vi "LTE_DPD_AMPM_EVM_ACP_DL.vi"() -> ()   [LabVIEW 2016]
doc: "This example illustrates how to use the RFmx SpecAn and LTE personalities together with the RFSG drivers to perform AMPM, EVM and ACP measurements with or without digital predistortion (DPD) of the LTE downlink waveform input to the DUT. \n\nDPD is a technique to optimize the operating point of power amplifiers and other non-linear RFIC devices. Power amplifiers are much more efficient if they operate near compression. However, compressing signal amplitudes can significantly deteriorate the amplified signal's quality both, in-band (e.g., EVM increases due to non-linear distortion of the signal's I/Q constellation) and out-of-band (e.g., ACP or SEM test fails due to spectral regrowth). With DPD, the original waveform is first pre-distorted in a way that matches the non-linear effects of the RFIC device before being fed through the device. The resulting output is a much cleaner amplified and/or filtered version of the original waveform. \n\nDifferent DPD models can be used to trade off performance with computational ease, with the Lookup-Table (LUT) model the simplest and the Generalized Memory Polynomial Model (GMP) the most complex. With a LUT, the DPD algorithm achieves gain and phase linearization on average. If you want to correct for memory effects - i.e., an output sample not only depends on the current input but also previous input samples; you will notice that a specific input power value translates into a range of gain and phase values - you would use one of the memory polynomial models. For these models, several parameters such as polynomial order and memory depth are available to fine-tune the model to the DUT behavior."
uses:
  Source/SG/Typedefs/Instrument Configuration.ctl
  <instrlib>/niRFSG/niRFSG.llb/niRFSG Ref Clock Sources.ctl
  Source/Common/Local Oscillator Sharing Mode.ctl
  Source/Common/SA Common Configuration.ctl
  <instrlib>/niRFSG/niRFSG.llb/niRFSG Exported Signal Destinations.ctl
  Source/SA/RFmxLTE/Typedefs/LTE Component Carrier Configuration.ctl
  Source/SA/RFmxLTE/Typedefs/LTE ModAcc Configuration.ctl
  Source/SA/RFmxLTE/Typedefs/LTE ACP Configuration.ctl
  Source/SA/RFmxLTE/Typedefs/LTE ACP Offset Results.ctl
  Source/SA/RFmxLTE/Typedefs/LTE ACP Component Carrier Results.ctl
  Source/SA/RFmxSpecAn/Typedefs/SpecAn AMPM Results.ctl
  Source/SA/RFmxSpecAn/Typedefs/SpecAn AMPM Configuration.ctl
  Source/Common/Waveform.ctl
  Source/Methods/RFmxDPD/Typedefs/Memory Polynomial Configuration.ctl
  Source/Methods/RFmxDPD/Typedefs/Common Configuration.ctl
  Source/SA/RFmxInstr/Typedefs/Instrument Configuration.ctl
  Source/Methods/RFmxDPD/Typedefs/Pre DPD Crest Factor Reduction Configuration.ctl
  Source/Methods/RFmxDPD/Typedefs/Pre DPD Crest Factor Reduction Carrier Channel.ctl
  Source/Methods/RFmxDPD/Typedefs/Apply DPD Crest Factor Reduction Configuration.ctl
  Source/Common/SA Auto Level Configuration.ctl
  <vilib>/RFmx/LTE/mx/RFmxLTE.llb/RFmxLTE ModAcc Fetch EVM per Subcarrier Trace.vi
  <vilib>/RFmx/LTE/mx/RFmxLTE.llb/RFmxLTE ACP Fetch Absolute Powers Trace.vi
  <vilib>/RFmx/LTE/mx/RFmxLTE.llb/RFmxLTE ACP Fetch Relative Powers Trace.vi
  <vilib>/RFmx/LTE/mx/RFmxLTE.llb/RFmxLTE ACP Fetch Spectrum.vi
  <vilib>/RFmx/LTE/mx/RFmxLTE.llb/RFmxLTE ModAcc Fetch PDSCH QPSK Constellation.vi
  <vilib>/RFmx/LTE/mx/RFmxLTE.llb/RFmxLTE ModAcc Fetch PDSCH 64 QAM Constellation.vi
  <vilib>/RFmx/LTE/mx/RFmxLTE.llb/RFmxLTE ModAcc Fetch PDSCH 16 QAM Constellation.vi
  <vilib>/RFmx/LTE/mx/RFmxLTE.llb/RFmxLTE ModAcc Fetch PDSCH 1024 QAM Constellation.vi
  <vilib>/RFmx/LTE/mx/RFmxLTE.llb/RFmxLTE ModAcc Fetch PDSCH 256 QAM Constellation.vi
  <vilib>/RFmx/SpecAn/mx/RFmxSpecAn.llb/RFmxSpecAn AMPM Fetch AM to PM Trace.vi
  <vilib>/RFmx/SpecAn/mx/RFmxSpecAn.llb/RFmxSpecAn AMPM Fetch AM to AM Trace.vi
  Source/SG/SG.lvlib
  Source/SA/RFmxLTE/RFmxLTE.lvlib
  Source/SA/RFmxSpecAn/RFmxSpecAn.lvlib
  Source/Methods/RFmxDPD/RFmxDPD.lvlib
  Source/SA/RFmxInstr/RFmxInstr.lvlib
  Source/Common/Common.lvlib
panel:
  in  "Error Tab Control":enum32{"Page 1", "Page 2"}(tab)
  out "error out":errorcluster
  in  "Display Tab Control":T1(tab)
  out "AM to PM Plot":T2(graph)
  out "AM to AM Plot":T3(graph)
  out "AMPM Measurement Results":T4 {"AM to PM Residual (deg)" format="%.2f"; "AM to AM Residual (dB)" format="%.2f"; "Mean RMS EVM (%)" format="%.2f"; "1 dB Compression Point (dBm)" format="%.2f"; "Mean Linear Gain (dB)" format="%.2f"}
  out "PDSCH QPSK Constellation Trace":cluster{"DMRS  Constellation":csg[]}[](graph)
  out "PDSCH 64 QAM Constellation Trace":cluster{"DMRS  Constellation":csg[]}[](graph)
  out "PDSCH 16 QAM Constellation Trace":cluster{"DMRS  Constellation":csg[]}[](graph)
  out "PDSCH 256 QAM Constellation Trace":cluster{"DMRS  Constellation":csg[]}[](graph)
  out "PDSCH 1024 QAM Constellation Trace":cluster{"DMRS  Constellation":csg[]}[](graph)
  out "EVM Per Subcarrier Trace":cluster{"x0":dbl, "dx":dbl, "y":sgl[]}(graph)
  out "ModAcc Results":T5
  out "ACP Results":T8
  out "Spectrum":cluster{"x0":dbl, "dx":dbl, "y":sgl[]}[](graph)
  out "Reference Waveform":cluster{"t0":dbl, "dt":dbl, "y":sgl[]}(graph)
  in  "Measurement Settings Tab Control":T9(tab)
  in  "RFmx SpecAn AMPM Configuration":T10={"Measurement Interval (s)"=0.0001, "DUT Average Input Power (dBm)"=-20.0, "Signal Type"=0, "Averaging Enabled"=0, "Averaging Count"=10, "Reference Waveform"={"Name"="Wfm", "Data"=refnum, "Signal Bandwidth (Hz)"=0.0, "PAPR (dB)"=0.0, "Burst Length (s)"=0.0, "Sample Rate"=0.0, "Burst Start Locations"=[], "Burst Stop Locations"=[], "Idle Duration Present?"=FALSE, "Runtime Scaling"=0.0, "Script"=""}} {"Reference Waveform"."Runtime Scaling" format="%#_6p"; "Reference Waveform"."Sample Rate" format="%#_6p"; "Reference Waveform"."Burst Length (s)" format="%#_6p"; "Reference Waveform"."PAPR (dB)" format="%.2f"; "Reference Waveform"."Signal Bandwidth (Hz)" format="%#_6p"; "Averaging Enabled" items=["False", "True"]; "Signal Type" items=["Modulated", "Tones"]; "DUT Average Input Power (dBm)" format="%.2f"; "Measurement Interval (s)" format="%.2p"}
  in  "Enable DPD":bool=TRUE
  in  "Common DPD Configuration":T12={"Measurement Interval (s)"=0.0001, "Signal Type"=0, "DUT Average Input Power (dBm)"=-15.0, "Synchronization Method"=1} {"Synchronization Method" items=["Direct"=1, "Alias Protected"=2]; "DUT Average Input Power (dBm)" format="%.2f"; "Signal Type" items=["Modulated", "Tones"]; "Measurement Interval (s)" format="%#.2p"}
  in  "Memory Polynomial Configuration":T13={"Correction Type"=0, "Number of Iterations"=1, " Order"=3, " Depth"=2, "Lead Order"=2, "Lag Order"=2, "Lead Memory Depth"=2, "Lag Memory Depth"=2, "Maximum Lead"=2, "Maximum Lag"=2} {"Number of Iterations" min=1; "Correction Type" items=["Magnitude and Phase", "Magnitude Only", "Phase Only"]}
  in  "Pre DPD Crest Factor Reduction":T14={"Enabled"=0, "Method"=0, "Max Iterations"=10, "Target PAPR (dB)"=8.0, "Shaping Factor"=5.0, "Shaping Threshold (dB)"=-5.0, "Window Type"=7, "Window Length"=10, "Filter Enabled"=0, "Carrier Channels"=[{"Offset (Hz)"=0.0, "Bandwidth (Hz)"=20000000.0}]} {"Carrier Channels"."Bandwidth (Hz)" format="%.2p"; "Carrier Channels"."Offset (Hz)" format="%.2p"; "Filter Enabled" items=["False", "True"]; "Window Type" items=["Flat Top"=1, "Hanning"=2, "Hamming"=3, "Gaussian"=4, "Blackman"=5, "Blackman-Harris"=6, "Kaiser-Bessel"=7]; "Method" items=["Clipping", "Peak Windowing", "Sigmoid"]; "Enabled" items=["False", "True"]}
  in  "Apply DPD Crest Factor Reduction":T16={"Enabled"=0, "Method"=0, "Max Iterations"=10, "Target PAPR Type"=0, "Target PAPR (dB)"=8.0, "Window Type"=7, "Window Length"=10, "Shaping Factor"=5.0, "Shaping Threshold (dB)"=-5.0} {"Target PAPR Type" items=["Input PAPR", "Custom"]; "Window Type" items=["Flat Top"=1, "Hanning"=2, "Hamming"=3, "Gaussian"=4, "Blackman"=5, "Blackman-Harris"=6, "Kaiser-Bessel"=7]; "Method" items=["Clipping", "Peak Windowing", "Sigmoid"]; "Enabled" items=["False", "True"]}
  in  "ModAcc Configuration":T17={"Synchronization Mode"=0, "Measurement Offset"=0, "Measurement Length"=1, "EVM Unit"=0, "Averaging Enabled"=0, "Averaging Count"=10} {"Averaging Enabled" items=["False", "True"]; "EVM Unit" items=["Percentage", "dB"]; "Synchronization Mode" items=["Frame", "Slot", "Marker"]}
  in  "ACP Configuration":T18={"Number of GSM Offsets"=0, "Number of UTRA Offsets"=2, "Number of EUTRA Offsets"=1, "Sweep Time Auto"=1, "Sweep Time Interval (s)"=0.001, "Averaging Enabled"=0, "Averaging Count"=10, "Averaging Type"=0, "RBW Auto"=1, "RBW (Hz)"=30000.0, "RBW Filter Type"=0} {"RBW Filter Type" items=["FFT Based", "Gaussian", "Flat"]; "RBW Auto" items=["False", "True"]; "Averaging Type" items=["RMS", "Log", "Scalar", "Max", "Min"]; "Averaging Enabled" items=["False", "True"]; "Sweep Time Auto" items=["False", "True"]}
  in  "Center Frequency (Hz)":dbl=1950000000.0 format="%.6p"
  in  "Resource Control":enum32{"RFSG", "RFSA", "LTE Signal"}(tab)
  in  "RFSG Resource Name":refnum<k15>="5840"
  in  "Reference Waveform File Path":path=path "C:/Users/Public/Documents/National Instruments/RFIC Test Software/Waveforms/LTE_FDD_DL_1x20MHz_TM11_OS4.tdms"
  in  "SG Configuration":T19={"SelectedPorts"="", "Reference Clock Source"="PXI_CLK", "Carrier Frequency (Hz)"=1000000000.0, "DUT Average Input Power (dBm)"=-10.0, "External Attenuation (dB)"=0.0, "LO Sharing Mode"=enum."Automatic"}
  in  "Marker Event Output Terminal":T22="PXI_Trig0"
  in  "RFSA Resource Name":refnum<k15>="5840"
  in  "Common Configuration":T23={"Center Frequency (Hz)"=1000000000.0, "Reference Level (dBm)"=0.0, "External Attenuation (dB)"=0.0, "Trigger Enabled"=TRUE, "Digital Trigger Source"="PXI_Trig0", "Trigger Delay (s)"=0.0, "Selected Ports"=""} {"Trigger Delay (s)" format="%.2p"; "External Attenuation (dB)" format="%.2f"; "Reference Level (dBm)" format="%.2f"; "Center Frequency (Hz)" format="%.6p"}
  in  "Instrument Configuration":T24={"LO Sharing Mode"=enum."Automatic", "Frequency Reference Source"="PXI_Clk"}
  in  "Auto Level Configuration":T25={"Enabled"=TRUE, "Measurement Interval (s)"=0.01} {"Measurement Interval (s)" min=1e-06 max=100.0 format="%.2p"}
  in  "Signal Configuration":T27={"Link Direction"=0, "Duplex Scheme"=0, "Uplink Downlink Config"=0, "Band"=1, "PUSCH Auto Resource Block Detection Enabled"=1, "Auto DMRS Detection Enabled"=0, "Downlink Auto Cell ID Detection Enabled"=1, "Component Carrier Configurations"=[{"Bandwidth (Hz)"=20000000.0, "Cell ID"=0, "PUSCH Modulation Type"=0, "PUSCH Resource Block Offset"=0, "PUSCH Number of Resource Blocks"=-1, "Downlink Test Model"=0}]} {"Downlink Auto Cell ID Detection Enabled" items=["False", "True"]; "Link Direction" items=["Downlink", "Uplink"]; "Auto DMRS Detection Enabled" items=["False", "True"]; "PUSCH Auto Resource Block Detection Enabled" items=["False", "True"]; "Component Carrier Configurations"."Downlink Test Model" items=["TM1.1", "TM1.2", "TM2", "TM 2a", "TM 3.1", "TM 3.2", "TM 3.3", "TM 3.1a"]; "Component Carrier Configurations"."PUSCH Modulation Type" items=["QPSK", "16 QAM", "64 QAM", "256 QAM", "1024 QAM"]; "Component Carrier Configurations"."Bandwidth (Hz)" items=["200.0 k"=200000.0, "1.4 M"=1400000.0, "3.0 M"=3000000.0, "5.0 M"=5000000.0, "10.0 M"=10000000.0, "15.0 M"=15000000.0, "20.0 M"=20000000.0]; "Uplink Downlink Config" items=["0", "1", "2", "3", "4", "5", "6"]; "Duplex Scheme" items=["FDD", "TDD", "LAA"]}
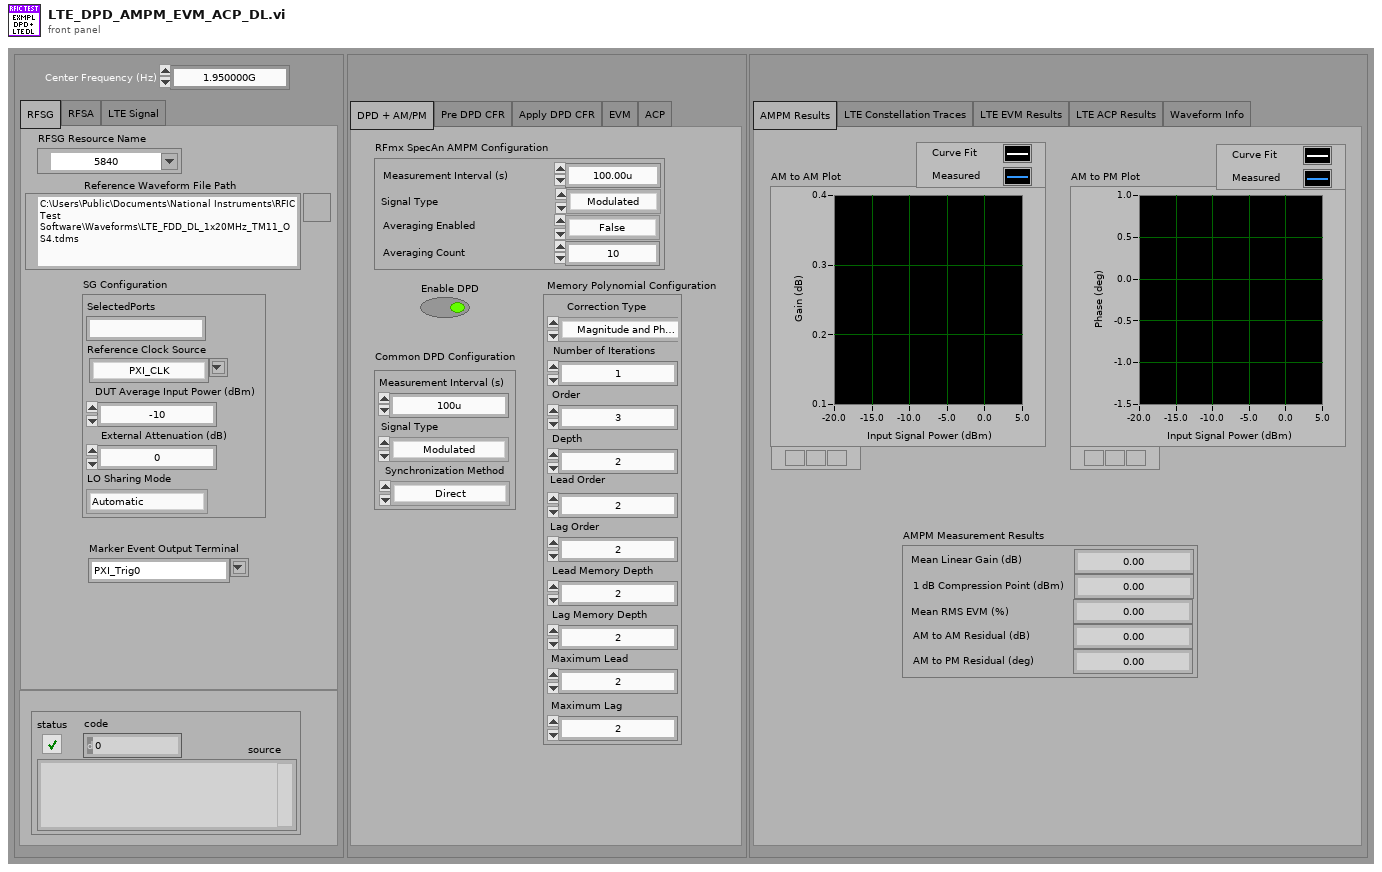
[diagram p1: front panel]
types:
  T1 = enum32{"AMPM Results", "LTE Constellation Traces", "LTE EVM Results", "LTE ACP Results", "Waveform Info"}
  T2 = cluster{"Input Powers (dBm)":sgl[], "Curve Fit AM to PM (dB)":sgl[]}[]
  T3 = cluster{"Input Powers (dBm)":sgl[], "Curve Fit AM to AM (dB)":sgl[]}[]
  T4 = typedef "RFmxSpecAn.lvlib/SpecAn AMPM Results.ctl" = cluster{"Mean Linear Gain (dB)":dbl, "1 dB Compression Point (dBm)":dbl, "Mean RMS EVM (%)":dbl, "AM to AM Residual (dB)":dbl, "AM to PM Residual (deg)":dbl}
  T5 = cluster{"Component Carrier Results":cluster{"Peak Composite EVM Subcarrier Index":i32, "Peak Composite EVM Symbol Index":i32, "Mean RMS Composite EVM":dbl, "Max Peak Composite EVM":dbl, "Mean Frequency Error (Hz)":dbl, "Peak Composite EVM Slot Index":i32}[]}
  T6 = typedef "RFmxLTE.lvlib/LTE ACP Offset Results.ctl" = cluster{"Lower Absolute Power (dBm)":dbl, "Upper Absolute Power (dBm)":dbl, "Lower Relative Power (dB)":dbl, "Upper Relative Power (dB)":dbl, "Frequency (Hz)":dbl, "Integration Bandwidth (Hz)":dbl}
  T7 = typedef "RFmxLTE.lvlib/LTE ACP Component Carrier Results.ctl" = cluster{"Absolute Power (dBm)":dbl, "Relative Power (dB)":dbl}
  T8 = cluster{"Offset Results":T6[], "Component Carrier Results":T7[]}
  T9 = enum32{"DPD + AM/PM", "Pre DPD CFR", "Apply DPD CFR", "EVM", "ACP"}
  T10 = typedef "RFmxSpecAn.lvlib/SpecAn AMPM Configuration.ctl" = cluster{"Measurement Interval (s)":dbl, "DUT Average Input Power (dBm)":dbl, "Signal Type":i32, "Averaging Enabled":i32, "Averaging Count":i32, "Reference Waveform":T11}
  T11 = typedef "Common.lvlib/Waveform.ctl" = cluster{"Name":string, "Data":refnum<data-value>, "Signal Bandwidth (Hz)":dbl, "PAPR (dB)":dbl, "Burst Length (s)":dbl, "Sample Rate":dbl, "Burst Start Locations":i32[], "Burst Stop Locations":i32[], "Idle Duration Present?":bool, "Runtime Scaling":dbl, "Script":string}
  T12 = typedef "RFmxDPD.lvlib/Common Configuration.ctl" = cluster{"Measurement Interval (s)":dbl, "Signal Type":i32, "DUT Average Input Power (dBm)":dbl, "Synchronization Method":i32}
  T13 = typedef "RFmxDPD.lvlib/Memory Polynomial Configuration.ctl" = cluster{"Correction Type":i32, "Number of Iterations":i32, " Order":i32, " Depth":i32, "Lead Order":i32, "Lag Order":i32, "Lead Memory Depth":i32, "Lag Memory Depth":i32, "Maximum Lead":i32, "Maximum Lag":i32}
  T14 = typedef "RFmxDPD.lvlib/Pre DPD Crest Factor Reduction Configuration.ctl" = cluster{"Enabled":i32, "Method":i32, "Max Iterations":i32, "Target PAPR (dB)":dbl, "Shaping Factor":dbl, "Shaping Threshold (dB)":dbl, "Window Type":i32, "Window Length":i32, "Filter Enabled":i32, "Carrier Channels":T15[]}
  T15 = typedef "RFmxDPD.lvlib/Pre DPD Crest Factor Reduction Carrier Channel.ctl" = cluster{"Offset (Hz)":dbl, "Bandwidth (Hz)":dbl}
  T16 = typedef "RFmxDPD.lvlib/Apply DPD Crest Factor Reduction Configuration.ctl" = cluster{"Enabled":i32, "Method":i32, "Max Iterations":i32, "Target PAPR Type":i32, "Target PAPR (dB)":dbl, "Window Type":i32, "Window Length":i32, "Shaping Factor":dbl, "Shaping Threshold (dB)":dbl}
  T17 = typedef "RFmxLTE.lvlib/LTE ModAcc Configuration.ctl" = cluster{"Synchronization Mode":i32, "Measurement Offset":i32, "Measurement Length":i32, "EVM Unit":i32, "Averaging Enabled":i32, "Averaging Count":i32}
  T18 = typedef "RFmxLTE.lvlib/LTE ACP Configuration.ctl" = cluster{"Number of GSM Offsets":i32, "Number of UTRA Offsets":i32, "Number of EUTRA Offsets":i32, "Sweep Time Auto":i32, "Sweep Time Interval (s)":dbl, "Averaging Enabled":i32, "Averaging Count":i32, "Averaging Type":i32, "RBW Auto":i32, "RBW (Hz)":dbl, "RBW Filter Type":i32}
  T19 = typedef "SG.lvlib/Instrument Configuration.ctl" = cluster{"SelectedPorts":string, "Reference Clock Source":T20, "Carrier Frequency (Hz)":dbl, "DUT Average Input Power (dBm)":dbl, "External Attenuation (dB)":dbl, "LO Sharing Mode":T21}
  T20 = typedef "niRFSG Ref Clock Sources.ctl" = string
  T21 = typedef "Common.lvlib/Local Oscillator Sharing Mode.ctl" = enum16{"Automatic", "None"}
  T22 = typedef "niRFSG Exported Signal Destinations.ctl" = string
  T23 = typedef "Common.lvlib/SA Common Configuration.ctl" = cluster{"Center Frequency (Hz)":dbl, "Reference Level (dBm)":dbl, "External Attenuation (dB)":dbl, "Trigger Enabled":bool, "Digital Trigger Source":string, "Trigger Delay (s)":dbl, "Selected Ports":string}
  T24 = typedef "RFmxInstr.lvlib/Instrument Configuration.ctl" = cluster{"LO Sharing Mode":T21, "Frequency Reference Source":string}
  T25 = typedef "Common.lvlib/SA Auto Level Configuration.ctl" = cluster{"Enabled":bool, "Measurement Interval (s)":dbl}
  T26 = typedef "RFmxLTE.lvlib/LTE Component Carrier Configuration.ctl" = cluster{"Bandwidth (Hz)":dbl, "Cell ID":i32, "PUSCH Modulation Type":i32, "PUSCH Resource Block Offset":i32, "PUSCH Number of Resource Blocks":i32, "Downlink Test Model":i32}
  T27 = cluster{"Link Direction":i32, "Duplex Scheme":i32, "Uplink Downlink Config":i32, "Band":i32, "PUSCH Auto Resource Block Detection Enabled":i32, "Auto DMRS Detection Enabled":i32, "Downlink Auto Cell ID Detection Enabled":i32, "Component Carrier Configurations":T26[]}
  T28 = enum16{"ACP", "CHP", "ModAcc", "OBW", "SEM", "PVT", "SlotPhase", "SlotPower"}[]
  T29 = enum16{"ACP", "CCDF", "CHP", "FCnt", "Harmonics", "OBW", "SEM", "Spectrum", "Spur", "TXP", "AMPM", "DPD", "IQ", "IM", "NF", "PhaseNoise", "PAVT"}[]
  T30 = cluster{"Reference Powers (dBm)":sgl[], "Curve Fit AM to AM (dB)":sgl[]}
  T31 = cluster{"Reference Powers (dBm)":sgl[], "Measured AM to AM (dB)":sgl[]}
  T32 = cluster{"Reference Powers (dBm)":sgl[], "Curve Fit AM to PM (deg)":sgl[]}
  T33 = cluster{"Reference Powers (dBm)":sgl[], "Measured AM to PM (deg)":sgl[]}
  T34 = cluster{"Reference Powers (dBm)":sgl[], "Measured AM to AM (dB)":sgl[]}[]
  T35 = cluster{"Reference Powers (dBm)":sgl[], "Measured AM to PM (deg)":sgl[]}[]
  T36 = typedef "RFmxLTE.lvlib/LTE ModAcc Results.ctl" = cluster{"Component Carrier Results":T37[]}
  T37 = typedef "RFmxLTE.lvlib/LTE ModAcc Component Carrier Results.ctl" = cluster{"Peak Composite EVM Subcarrier Index":i32, "Peak Composite EVM Symbol Index":i32, "Mean RMS Composite EVM":dbl, "Max Peak Composite EVM":dbl, "Mean Frequency Error (Hz)":dbl, "Peak Composite EVM Slot Index":i32}
  T38 = typedef "RFmxLTE.lvlib/LTE ACP Results.ctl" = cluster{"Offset Results":T6[], "Component Carrier Results":T7[]}
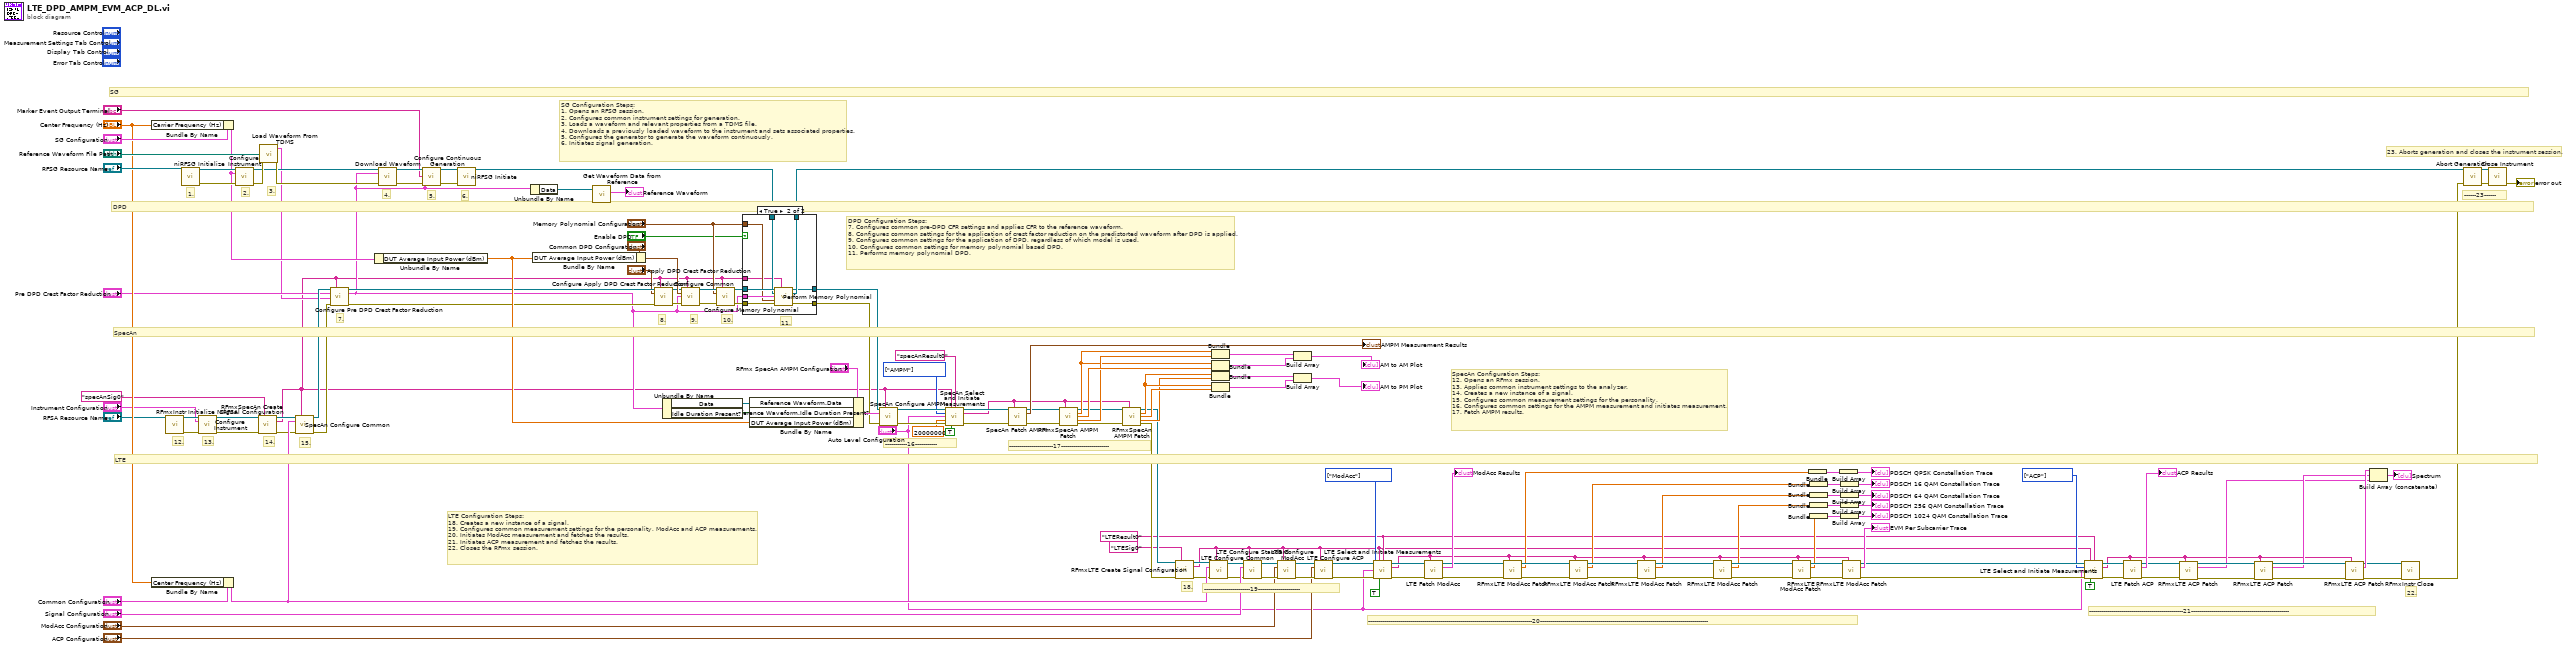
[diagram p0: block diagram]
diagram:
  w5 = "LTEResult0"
  w22 = T28 [enum."ACP"] items=["ACP", "CHP", "ModAcc", "OBW", "SEM", "PVT", "SlotPhase", "SlotPower"] ("Measurements")
  w28 = T28 [enum."ModAcc"] items=["ACP", "CHP", "ModAcc", "OBW", "SEM", "PVT", "SlotPhase", "SlotPower"] ("Measurements")
  w35 = T29 [enum."AMPM"] items=["ACP", "CCDF", "CHP", "FCnt", "Harmonics", "OBW", "SEM", "Spectrum", "Spur", "TXP", "AMPM", "DPD", "IQ", "IM", "NF", "PhaseNoise", "PAVT"] ("Measurements")
  # "23. Aborts generation and closes the instrument session."
  # "------23------"
  # "22."
  # "-----------------------------------------------21-------------------------------------------------"
  # "LTE Configuration Steps:\n18. Creates a new instance of a signal.\n19. Configures common measurement settings for the personality, ModAcc and ACP measurements.\n20. Initiates ModAcc measurement and fetches the results. \n21. Initiates ACP measurement and fetches the results.\n22. Closes the RFmx session."
  # "----------------------------------------------------------------------------------20------------------------------------------------------------------------------------"
  # "-----------------------19---------------------"
  # "18."
  # "SpecAn Configuration Steps:\n12. Opens an RFmx session.\n13. Applies common instrument settings to the analyzer.\n14. Creates a new instance of a signal.\n15. Configures common measurement settings for the personality.\n16. Configures common settings for the AMPM measurement and initiates measurement.\n17. Fetch AMPM results."
  # "----------------------17------------------------"
  # "-----------16-----------"
  # "15."
  # "14."
  # "13."
  # "12."
  # "DPD Configuration Steps:\n7. Configures common pre-DPD CFR settings and applies CFR to the reference waveform.\n8. Configures common settings for the application of crest factor reduction on the predistorted waveform after DPD is applied.\n9. Configures common settings for the application of DPD, regardless of which model is used. \n10. Configures common settings for memory polynomial based DPD.\n11. Performs memory polynomial DPD."
  # "11."
  # "10."
  # "9."
  # "8."
  # "7."
  # "SG Configuration Steps:\n1. Opens an RFSG session.\n2. Configures common instrument settings for generation.\n3. Loads a waveform and relevant properties from a TDMS file.\n4. Downloads a previously loaded waveform to the instrument and sets associated properties.\n5. Configures the generator to generate the waveform continuously.\n6. Initiates signal generation."
  # "6."
  # "5."
  # "4."
  # "3."
  # "2."
  # "1."
  # "SpecAn"
  # "LTE"
  # "DPD"
  # "SG"
  n1 = Bundle By Name(cluster="SG Configuration", "Carrier Frequency (Hz)"="Center Frequency (Hz)") -> (w146:T19)
  n2 = Bundle By Name(cluster="Common Configuration", "Center Frequency (Hz)"="Center Frequency (Hz)") -> (w56:T23)
  n3 = call <vilib>:"RFmxInstr Initialize NIRFSA.vi"("Resource Name"="RFSA Resource Name") -> ("Instrument Handle Out"=w55:refnum<k21>, "error out"=w54:errorcluster)  [unwired: 12 in, 1 out]
  n4 = call <instrlib>:"niRFSG Initialize.vi"("resource name"="RFSG Resource Name") -> ("instrument handle"=w156:refnum<k15>, "error out"=w155:errorcluster)  [unwired: 13 in]
  n5 = call "Configure Instrument.vi"("Instrument Handle In"=w55, "Instrument Configuration"="Instrument Configuration", "error in (no error)"=w54) -> ("Instrument Handle Out"=w17:refnum<k21>, "error out"=w14:errorcluster)  [unwired: 11 in]
  n6 = call "Configure Instrument.vi"("RFSG Session In"=w156, "SG Configuration"=w146, "error in (no error)"=w155) -> ("RFSG Session Out"=w157:refnum<k15>, "error out"=w159:errorcluster)  [unwired: 11 in]
  n7 = call <vilib>:"RFmxSpecAn Create Signal Configuration.vi"("Instrument Handle In"=w17, "Signal Name"="specAnSig0", "error in (no error)"=w14) -> ("Instrument Handle Out"=w16:refnum<k21>, "Selector String Out"=w12:string, "error out"=w15:errorcluster)  [unwired: 10 in]
  n8 = call "Load Waveform From TDMS.vi"("TDMS File Path"="Reference Waveform File Path", "error in (no error)"=w159) -> ("Waveform"=w40:T11, "error out"=w158:errorcluster)  [unwired: 12 in]
  n9 = call "SpecAn Configure Common.vi"("RFmx Handle In"=w16, "Selector String"=w12, "Common Configuration"=w56, "error in (no error)"=w15) -> ("RFmx Handle Out"=w48:refnum<k21>, "error out"=w18:errorcluster)  [unwired: 10 in]
  n10 = call "Configure Pre DPD Crest Factor Reduction.vi"("Instrument Handle In"=w48, "Selector String"=w12, "Pre DPD Crest Factor Reduction Configuration"="Pre DPD Crest Factor Reduction", "Reference Waveform"=w40, "error in (no error)"=w18) -> ("Instrument Handle Out"=w52:refnum<k21>, "Pre DPD CFR Waveform"=w19:T11, "error out"=w51:errorcluster)  [unwired: 8 in]
  n11 = Unbundle By Name(w146) -> ("DUT Average Input Power (dBm)"=w62:dbl)
  n12 = call "Download Waveform.vi"("RFSG handle"=w157, "Waveform In"=w19, "error in (no error)"=w158) -> ("RFSG handle out"=w153:refnum<k15>, "error out"=w152:errorcluster)  [unwired: 11 in]
  n13 = call "Configure Continuous Generation.vi"("RFSG handle"=w153, "Waveform in"=w19, "Waveform Start Trigger Export"="Marker Event Output Terminal", "error in"=w152) -> ("RFSG handle out"=w154:refnum<k15>, "error out"=w68:errorcluster)  [unwired: 9 in, 1 out]
  n14 = call <instrlib>:"niRFSG Initiate.vi"("instrument handle"=w154, "error in"=w68) -> ("instrument handle out"=w61:refnum<k15>)  [unwired: 12 in, 1 out]
  n15 = Unbundle By Name(w19) -> ("Data"=w42:refnum<data-value>)
  n16 = Bundle By Name(cluster="Common DPD Configuration", "DUT Average Input Power (dBm)"=w62) -> (w63:T12)
  n17 = call "Get Waveform Data from Reference.vi"("Waveform Data Reference"=w42) -> ("Waveform Data"=→"Reference Waveform":cluster{"t0":dbl, "dt":dbl, "y":csg[]})  [unwired: 13 in, 1 out]
  n18 = call "Configure Apply DPD Crest Factor Reduction.vi"("Instrument Handle In"=w52, "Selector String"=w12, "Apply DPD Crest Factor Reduction Configuration"="Apply DPD Crest Factor Reduction", "error in (no error)"=w51) -> ("Instrument Handle Out"=w50:refnum<k21>, "error out"=w49:errorcluster)  [unwired: 10 in]
  n19 = Unbundle By Name(w19) -> ("Data"=w148:refnum<data-value>, "Idle Duration Present?"=w147:bool)
  n20 = call "Configure Common.vi"("Instrument Handle In"=w50, "Selector String"=w12, "Common Configuration"=w63, "Reference Waveform"=w19, "error in (no error)"=w49) -> ("Instrument Handle Out"=w70:refnum<k21>, "error out"=w69:errorcluster)  [unwired: 9 in]
  n21 = call "Configure Memory Polynomial.vi"("Instrument Handle In"=w70, "Selector String"=w12, "Memory Polynomial Configuration"="Memory Polynomial Configuration", "error in (no error)"=w69) -> ("Instrument Handle Out"=w71:refnum<k21>, "error out"=w72:errorcluster)  [unwired: 10 in]
  n22 = case shown="True" "Enable DPD" {
    tunnel: w71 -> [w161 w171]
    tunnel: [w160 w170] -> w57
    tunnel: "Memory Polynomial Configuration" -> [_ w164]
    tunnel: w19 -> [_ w169]
    tunnel: w61 -> [w162 w168]
    tunnel: [w162 w167] -> w60
    tunnel: [w161 w166] -> w58
    tunnel: w72 -> [w160 w165]
    tunnel: w12 -> [_ w163]
    frame False {
    }
    frame True {
      n23 = call "Perform Memory Polynomial.vi"("RFmx Instrument Handle In"=w171, "Selector String"=w163, "RFSG Instrument Handle In"=w168, "Reference Waveform"=w169, "Memory Polynomial Configuration"=w164, "error in (no error)"=w165) -> ("RFmx Instrument Handle Out"=w166:refnum<k21>, "RFSG Instrument Handle Out"=w167:refnum<k15>, "error out"=w170:errorcluster)  [unwired: 6 in, 1 out]
    }
  }
  n24 = Bundle By Name(cluster="RFmx SpecAn AMPM Configuration", "Reference Waveform.Data"=w148, "Reference Waveform.Idle Duration Present?"=w147, "DUT Average Input Power (dBm)"=w62) -> (w90:T10)
  n25 = call "SpecAn Configure AMPM.vi"("RFmx Handle In"=w58, "Selector String"=w12, "RFmx SpecAn AMPM Configuration"=w90, "error in (no error)"=w57) -> ("RFmx Handle Out"=w39:refnum<k21>, "error out"=w38:errorcluster)  [unwired: 10 in]
  n26 = call "SpecAn Select and Initiate Measurements.vi"("Instrument Handle In"=w39, "Selector String"=w12, "Result Name"="specAnResult0", "Measurements"=w35, "Auto Level Configuration"="Auto Level Configuration", "Auto Level Bandwidth (Hz)"=20000000.0, "error in (no error)"=w38, "Enable All Traces (F)"=TRUE) -> ("Instrument Handle Out"=w36:refnum<k21>, "Selector String Out"=w1:string, "error out"=w37:errorcluster)  [unwired: 5 in]
  n27 = call "SpecAn Fetch AMPM.vi"("RFmx Handle In"=w36, "Selector String"=w1, "error in (no error)"=w37) -> ("RFmx Handle Out"=w76:refnum<k21>, "AMPM Results"=→"AMPM Measurement Results":T4, "error out"=w75:errorcluster)  [unwired: 10 in]
  n28 = call-poly <vilib>:"RFmxSpecAn AMPM Fetch.vi"("Instrument Handle In"=w76, "Selector String"=w1, "error in (no error)"=w75) -> ("Instrument Handle Out"=w82:refnum<k21>, "Reference Powers (dBm)"=w86:sgl[], "Measured AM to AM (dB)"=w88:sgl[], "Curve Fit AM to AM (dB)"=w87:sgl[], "error out"=w81:errorcluster)  [unwired: 8 in]
  n29 = call-poly <vilib>:"RFmxSpecAn AMPM Fetch.vi"("Instrument Handle In"=w82, "Selector String"=w1, "error in (no error)"=w81) -> ("Instrument Handle Out"=w11:refnum<k21>, "Reference Powers (dBm)"=w85:sgl[], "Measured AM to PM (deg)"=w84:sgl[], "Curve Fit AM to PM (deg)"=w83:sgl[], "error out"=w9:errorcluster)  [unwired: 8 in]
  n30 = call <vilib>:"RFmxLTE Create Signal Configuration.vi"("Instrument Handle In"=w11, "Signal Name"="LTESig0", "error in (no error)"=w9) -> ("Instrument Handle Out"=w10:refnum<k21>, "Selector String Out"=w4:string, "error out"=w8:errorcluster)  [unwired: 10 in]
  n31 = call "LTE Configure Common.vi"("RFmx Handle In"=w10, "Selector String"=w4, "Common Configuration"=w56, "error in (no error)"=w8) -> ("RFmx Handle Out"=w67:refnum<k21>, "error out"=w66:errorcluster)  [unwired: 10 in]
  n32 = Bundle("Reference Powers (dBm)"=w86, "Curve Fit AM to AM (dB)"=w87) -> (w80:T30)  [unwired: 1 in]
  n33 = Bundle("Reference Powers (dBm)"=w86, "Measured AM to AM (dB)"=w88) -> (w79:T31)  [unwired: 1 in]
  n34 = Bundle("Reference Powers (dBm)"=w85, "Curve Fit AM to PM (deg)"=w83) -> (w77:T32)  [unwired: 1 in]
  n35 = Bundle("Reference Powers (dBm)"=w85, "Measured AM to PM (deg)"=w84) -> (w78:T33)  [unwired: 1 in]
  n36 = call "LTE Configure Standard.vi"("RFmx Handle In"=w67, "Selector String"=w4, "LTE Standard Configuration"="Signal Configuration", "error in (no error)"=w66) -> ("RFmx Handle Out"=w136:refnum<k21>, "error out"=w137:errorcluster)  [unwired: 10 in]
  n37 = call "LTE Configure ModAcc.vi"("RFmx Handle In"=w136, "Selector String"=w4, "ModAcc Configuration"="ModAcc Configuration", "error in (no error)"=w137) -> ("RFmx Handle Out"=w135:refnum<k21>, "error out"=w134:errorcluster)  [unwired: 10 in]
  n38 = Build Array(w80, w79) -> (→"AM to AM Plot":T34)
  n39 = Build Array(w77, w78) -> (→"AM to PM Plot":T35)
  n40 = call "LTE Configure ACP.vi"("RFmx Handle In"=w135, "Selector String"=w4, "ACP Configuration"="ACP Configuration", "error in (no error)"=w134) -> ("RFmx Handle Out"=w32:refnum<k21>, "error out"=w30:errorcluster)  [unwired: 10 in]
  n41 = call "LTE Select and Initiate Measurements.vi"("Instrument Handle In"=w32, "Selector String"=w4, "Result Name"=w5, "Measurements"=w28, "Auto Level Configuration"="Auto Level Configuration", "error in (no error)"=w30, "Enable All Traces (F)"=TRUE) -> ("Instrument Handle Out"=w31:refnum<k21>, "Selector String Out"=w6:string, "error out"=w29:errorcluster)  [unwired: 6 in]
  n42 = call "LTE Fetch ModAcc.vi"("RFmx Handle In"=w31, "Selector String"=w6, "error in (no error)"=w29) -> ("RFmx Handle Out"=w117:refnum<k21>, "ModAcc Results"=→"ModAcc Results":T36, "error out"=w118:errorcluster)  [unwired: 10 in]
  n43 = call-poly <vilib>:"RFmxLTE ModAcc Fetch.vi"("Instrument Handle In"=w117, "Selector String"=w6, "error in (no error)"=w118) -> ("Instrument Handle Out"=w116:refnum<k21>, "PDSCH QPSK Constellation"=w101:csg[], "error out"=w115:errorcluster)  [unwired: 10 in]
  n44 = call-poly <vilib>:"RFmxLTE ModAcc Fetch.vi"("Instrument Handle In"=w116, "Selector String"=w6, "error in (no error)"=w115) -> ("Instrument Handle Out"=w114:refnum<k21>, "PDSCH 16 QAM Constellation"=w99:csg[], "error out"=w113:errorcluster)  [unwired: 10 in]
  n45 = call-poly <vilib>:"RFmxLTE ModAcc Fetch.vi"("Instrument Handle In"=w114, "Selector String"=w6, "error in (no error)"=w113) -> ("Instrument Handle Out"=w112:refnum<k21>, "PDSCH 64 QAM Constellation"=w94:csg[], "error out"=w111:errorcluster)  [unwired: 10 in]
  n46 = call-poly <vilib>:"RFmxLTE ModAcc Fetch.vi"("Instrument Handle In"=w112, "Selector String"=w6, "error in (no error)"=w111) -> ("Instrument Handle Out"=w110:refnum<k21>, "PDSCH 256 QAM Constellation"=w93:csg[], "error out"=w108:errorcluster)  [unwired: 10 in]
  n47 = call-poly <vilib>:"RFmxLTE ModAcc Fetch.vi"("Instrument Handle In"=w110, "Selector String"=w6, "error in (no error)"=w108) -> ("Instrument Handle Out"=w109:refnum<k21>, "1024 QAM Constellation"=w92:csg[], "error out"=w107:errorcluster)  [unwired: 10 in]
  n48 = Bundle("PDSCH QPSK Constellation"=w101) -> (w106:cluster{"PDSCH QPSK Constellation":csg[]})  [unwired: 1 in]
  n49 = Bundle("PDSCH 16 QAM Constellation"=w99) -> (w105:cluster{"PDSCH 16 QAM Constellation":csg[]})  [unwired: 1 in]
  n50 = Bundle("PDSCH 64 QAM Constellation"=w94) -> (w104:cluster{"PDSCH 64 QAM Constellation":csg[]})  [unwired: 1 in]
  n51 = Bundle("PDSCH 256 QAM Constellation"=w93) -> (w103:cluster{"PDSCH 256 QAM Constellation":csg[]})  [unwired: 1 in]
  n52 = Bundle("1024 QAM Constellation"=w92) -> (w102:cluster{"1024 QAM Constellation":csg[]})  [unwired: 1 in]
  n53 = Build Array(w106) -> (→"PDSCH QPSK Constellation Trace":cluster{"PDSCH QPSK Constellation":csg[]}[])
  n54 = Build Array(w105) -> (→"PDSCH 16 QAM Constellation Trace":cluster{"PDSCH 16 QAM Constellation":csg[]}[])
  n55 = Build Array(w104) -> (→"PDSCH 64 QAM Constellation Trace":cluster{"PDSCH 64 QAM Constellation":csg[]}[])
  n56 = Build Array(w103) -> (→"PDSCH 256 QAM Constellation Trace":cluster{"PDSCH 256 QAM Constellation":csg[]}[])
  n57 = Build Array(w102) -> (→"PDSCH 1024 QAM Constellation Trace":cluster{"1024 QAM Constellation":csg[]}[])
  n58 = call-poly <vilib>:"RFmxLTE ModAcc Fetch.vi"("Instrument Handle In"=w109, "Selector String"=w6, "error in (no error)"=w107) -> ("Instrument Handle Out"=w26:refnum<k21>, "Mean RMS EVM per Subcarrier (% or dB)"=→"EVM Per Subcarrier Trace":cluster{"x0":dbl, "dx":dbl, "y":sgl[]}, "error out"=w24:errorcluster)  [unwired: 10 in]
  n59 = call "LTE Select and Initiate Measurements.vi"("Instrument Handle In"=w26, "Selector String"=w4, "Result Name"=w5, "Measurements"=w22, "Auto Level Configuration"="Auto Level Configuration", "error in (no error)"=w24, "Enable All Traces (F)"=TRUE) -> ("Instrument Handle Out"=w25:refnum<k21>, "Selector String Out"=w3:string, "error out"=w23:errorcluster)  [unwired: 6 in]
  n60 = call "LTE Fetch ACP.vi"("RFmx Handle In"=w25, "Selector String"=w3, "error in (no error)"=w23) -> ("RFmx Handle Out"=w121:refnum<k21>, "ACP Results"=→"ACP Results":T38, "error out"=w120:errorcluster)  [unwired: 10 in]
  n61 = call-poly <vilib>:"RFmxLTE ACP Fetch.vi"("Instrument Handle In"=w121, "Selector String"=w3, "error in (no error)"=w120) -> ("Instrument Handle Out"=w129:refnum<k21>, "Absolute Powers (dBm)"=w123:cluster{"x0":dbl, "dx":dbl, "y":sgl[]}[], "error out"=w127:errorcluster)  [unwired: 10 in]
  n62 = call-poly <vilib>:"RFmxLTE ACP Fetch.vi"("Instrument Handle In"=w129, "Selector String"=w3, "error in (no error)"=w127) -> ("Instrument Handle Out"=w128:refnum<k21>, "Relative Powers (dB)"=w124:cluster{"x0":dbl, "dx":dbl, "y":sgl[]}[], "error out"=w126:errorcluster)  [unwired: 10 in]
  n63 = call-poly <vilib>:"RFmxLTE ACP Fetch.vi"("Instrument Handle In"=w128, "Selector String"=w3, "error in (no error)"=w126) -> ("Instrument Handle Out"=w44:refnum<k21>, "Spectrum (dBm)"=w125:cluster{"x0":dbl, "dx":dbl, "y":sgl[]}, "error out"=w45:errorcluster)  [unwired: 10 in]
  n64 = Build Array (concatenate)(w125, w124, w123) -> (→"Spectrum":cluster{"x0":dbl, "dx":dbl, "y":sgl[]}[])
  n65 = call <vilib>:"RFmxInstr Close.vi"("Instrument Handle In"=w44, "error in (no error)"=w45) -> ("error out"=w43:errorcluster)  [unwired: 13 in]
  n66 = call "Abort Generation.vi"("RFSG handle"=w60, "error in (no error)"=w43) -> ("RFSG handle out"=w140:refnum<k15>, "error out"=w141:errorcluster)  [unwired: 12 in]
  n67 = call "Close Instrument.vi"("RFSG Handle"=w140, "error in (no error)"=w141) -> ("error out"=→"error out":errorcluster)  [unwired: 13 in]
